vi "dist_to_rpm.vi"(10 "Distance (in)":dbl) -> (2 "RPM":dbl)   [LabVIEW 2020]
panel:
  in  "c":dbl=3931.46898
  in  "b":dbl=10.7310594
  in  "a":dbl=0.0613687515
  # "ax^2+bx+c"
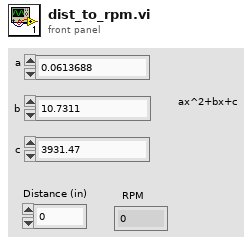
[diagram p1: front panel]
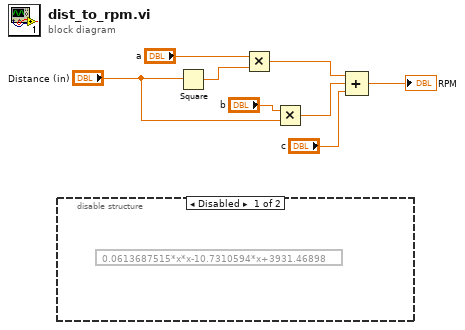
[diagram p0: block diagram]
diagram:
  n1 = disable-structure shown="Disabled" {
    frame Disabled {
      n2 = expression code="0.0613687515*x*x-10.7310594*x+3931.46898"() -> ()  [unwired: 1 in, 1 out]
    }
    frame Enabled {
    }
  }
  n3 = Square(x="Distance (in)") -> (x^2=w8:dbl)
  n4 = Multiply(x="a", y=w8) -> (x*y=w4:dbl)
  n5 = Multiply(x="b", y="Distance (in)") -> (x*y=w3:dbl)
  n6 = Compound Arithmetic op=ADD(w4, w3, "c") -> (→"RPM":dbl)
